vi "MoveDir.vi"(8 "Type":enum16{"Random", "Simple"}(ring)=enum."Simple", 10 "View":i32[](array[numeric]) caption="View (Team Index, -1: empty)", 11 "Atom In":refnum<class "Atom.lvclass">) -> (1 "ValidDir":bool, 2 "Direction":T1=enum."N", 3 "Atom Out":refnum<class "Atom.lvclass">)   [LabVIEW 2020, in "Atom.lvclass"]
uses:
  Atom.lvclass
  Type Defs/Direction Enum.ctl
  Type Defs/SB Type Defs.lvlib
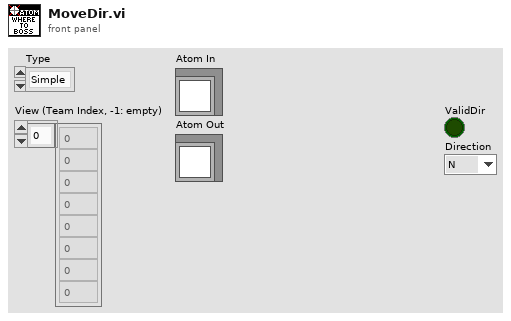
[diagram p1: front panel]
types:
  T1 = typedef "SB Type Defs.lvlib/Direction Enum.ctl" = enum16{"NW", "N", "NE", "E", "SE", "S", "SW", "W"}
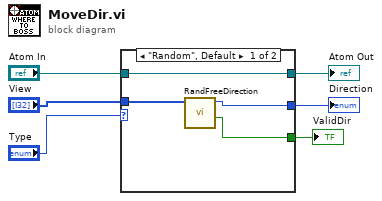
[diagram p0: block diagram]
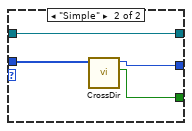
[diagram p2: hidden frame]
diagram:
  n1 = case shown="\"Random\", Default" "Type" {
    tunnel: "View" -> [w10 w14]
    tunnel: [w9 w13] -> w4
    tunnel: [w8 w12] -> w3
    tunnel: "Atom In" -> [w7 w11]
    tunnel: [w7 w11] -> w1
    frame "Random", Default {
      n2 = call "RandFreeDirection.vi"("View"=w10) -> ("Free space?"=w8:bool, "Direction"=w9:T1)  [unwired: 9 in]
    }
    frame "Simple" {
      n3 = call "CrossDir.vi"("View"=w14) -> ("ValidDir"=w12:bool, "Direction"=w13:T1)  [unwired: 9 in]
    }
  }
  "ValidDir" <- w3
  "Direction" <- w4
  "Atom Out" <- w1
